vi "Kommandos verwalten.vi"(6 "Aktionen":T1, 9 "NEUE Kommandos":string[](array[string])=["AKON", "AKON", "AKON", "AKON", "AKON", "AKON", "AKON", "AKON", "AKON", "AKON"], 11 "neues Kommando":string) -> (0 "Zeitstempeln":timestamp[](array[timestamp]), 1 "NEUE Kommandos":string[](array[string])=["ASTZ", "AKON", "AKON", "AKON", "AKON", "AKON", "AKON", "AKON", "AKON", "AKON", "AKON"], 3 "Kommandos":string[](array[string]))   [LabVIEW 2020, in "FT-IR.lvlib" / "AK-Interface.lvlib"]
uses:
  AK-Interface.lvlib
  Kommandos verwalten Aktionen.ctl
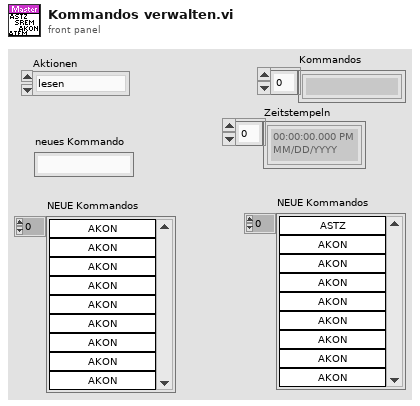
[diagram p1: front panel]
types:
  T1 = typedef "FT-IR.lvlib/AK-Interface.lvlib/Kommandos verwalten Aktionen.ctl" = enum16{"lesen", "setzen Ende", "setzen Pos1", "senden", "initalisieren", "prüfen", "Kommandos"}
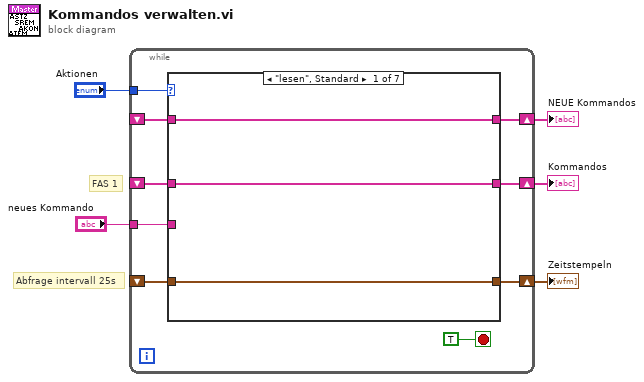
[diagram p0: block diagram]
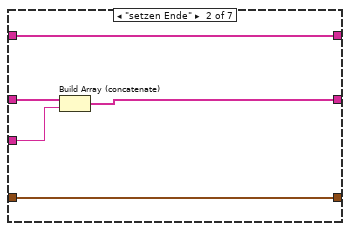
[diagram p2: hidden frame]
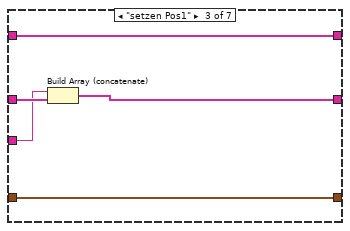
[diagram p3: hidden frame]
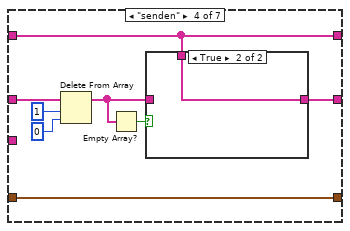
[diagram p4: hidden frame]
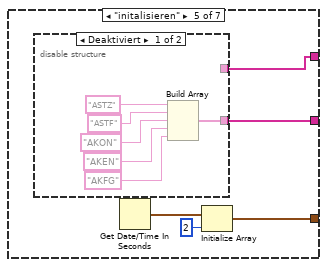
[diagram p6: hidden frame]
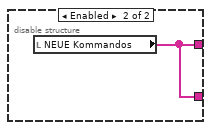
[diagram p7: hidden frame]
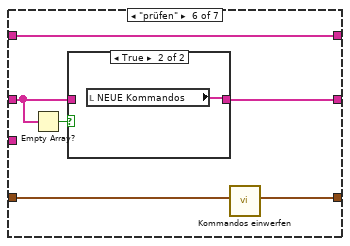
[diagram p8: hidden frame]
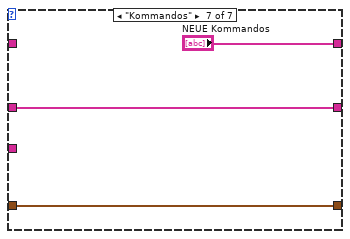
[diagram p10: hidden frame]
diagram:
  # "FAS 1"
  # "Abfrage intervall 25s"
  n1 = while {
    tunnel: "Aktionen" -> [w14]
    shift-right: [w12] -> w3
    shift-left: _ -> [w13]
    tunnel: "neues Kommando" -> [w11]
    shift-right: [w9] -> w2
    shift-left: _ -> [w8]
    shift-right: [w7] -> w1
    shift-left: _ -> [w6]
    stop <- TRUE stop-if-true
    n2 = case shown="\"lesen\", Standard" w14 {
      tunnel: w13 -> [w17 w22 w26 w35 _ w52 w59]
      tunnel: [w17 w21 w25 w29 w39 w50 w59] -> w12
      tunnel: w11 -> [_ w20 w24 _ _ _ _]
      tunnel: [w16 w19 w27 w34 w40 w54 w58] -> w9
      tunnel: w8 -> [w16 w19 w27 w34 _ w55 w58]
      tunnel: [w15 w18 w23 w28 w38 w51 "NEUE Kommandos"] -> w7
      tunnel: w6 -> [w15 w18 w23 w28 _ w51 _]
      frame "lesen", Default {
      }
      frame "setzen Ende" {
        n3 = Build Array (concatenate)(w22, w20) -> (w21:string[])
      }
      frame "setzen Pos1" {
        n4 = Build Array (concatenate)(w24, w26) -> (w25:string[])
      }
      frame "senden" {
        n5 = Delete From Array(array=w35, length=1 ("Länge"), index=0 ("Index")) -> (array with subset deleted=w30:string[])  [unwired: 1 out]
        n6 = Empty Array?(array=w30) -> (empty?=w31:bool)
        n7 = case shown="True" w31 {
          tunnel: w30 -> [w36 _]
          tunnel: [w36 w37] -> w29
          tunnel: w28 -> [_ w37]
          frame False {
          }
          frame True {
          }
        }
      }
      frame "initalisieren" {
        n8 = disable-structure shown="Deaktiviert" {
          disable-tunnel: [w44 w49] -> w39
          disable-tunnel: [_ w49] -> w38
          frame Disabled {
            n9 = Build Array("ASTZ", "ASTF", "AKON", "AKEN", "AKFG") -> (w44:string[])
          }
          frame Enabled {
            n10 = local read "NEUE Kommandos"() -> (w49:string[])
          }
        }
        n11 = Get Date/Time In Seconds() -> (seconds since 1Jan1904=w42:timestamp)
        n12 = Initialize Array(w42, 2 ("Dimension")) -> (w40:timestamp[])
      }
      frame "prüfen" {
        n13 = Empty Array?(array=w52) -> (empty?=w53:bool)
        n14 = case shown="True" w53 {
          tunnel: w52 -> [w56 _]
          tunnel: [w56 w57] -> w50
          frame False {
          }
          frame True {
            n15 = local read "NEUE Kommandos"() -> (w57:string[])
          }
        }
        n16 = call "Kommandos einwerfen.vi"("Zeitstempeln"=w55) -> ("Zeitstempeln"=w54:timestamp[])  [unwired: 9 in, 1 out]
      }
      frame "Kommandos" {
      }
    }
  }
  "Kommandos" <- w3
  "Zeitstempeln" <- w2
  "NEUE Kommandos" <- w1
